vi "UTIL_Add array to queue v1_0_0.vi"(6 "Queue elements":string[](array[string]), 7 "Flush (f)":bool, 8 "error in (no error)":errorcluster, 9 "Queue position":enum16{"top", "bottom"}(ring)=enum."bottom", 11 "Queue in":refnum<queue>) -> (0 "error out":errorcluster, 3 "Queue out":refnum<queue>)   [LabVIEW 2015]
doc: "UTIL_Add array to queue v1_0_0.vi\n\nIf flush queue first boolean is true it revoves any existing queue elements from the queue array. If false, Items already existing on the queue array will remain.\n\nAny items that exist in the Queue elements control are then added to either the top or bottom of the array depending on the Queue position control\n\nCreated 2006 by\nJim Tersigni\nNational Analytics\n970-397-0764"
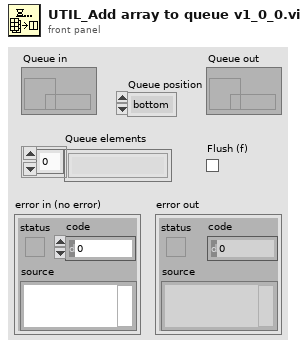
[diagram p1: front panel]
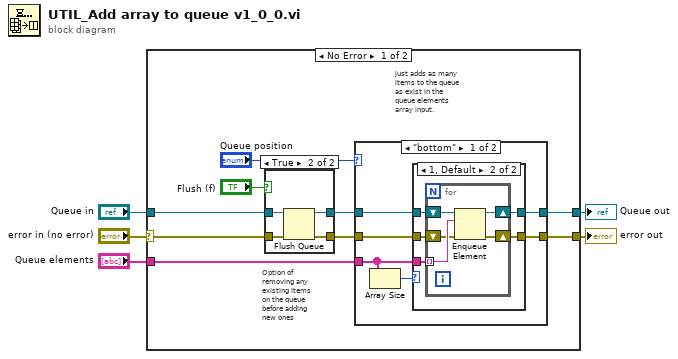
[diagram p0: block diagram]
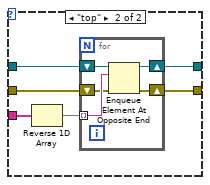
[diagram p4: hidden frame]
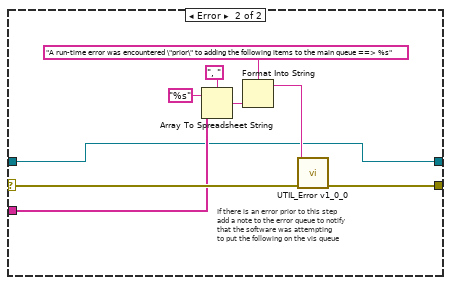
[diagram p5: hidden frame]
diagram:
  n1 = case shown="No Error" "error in (no error)" {
    selector: "error in (no error)" -> [w8 w58]
    tunnel: "Queue in" -> [w14 w51]
    tunnel: [w13 w57] -> w4
    tunnel: "Queue elements" -> [w7 w53]
    tunnel: [w6 w51] -> w1
    frame No Error {
      # "just adds as many\nitems to the queue\nas exist in the\nqueue elements\narray input."
      # "Option of \nremoving any\nexisting items\non the queue\nbefore adding \nnew ones"
      n2 = case shown="True" "Flush (f)" {
        tunnel: w8 -> [w15 w20]
        tunnel: [w15 w19] -> w10
        tunnel: [w16 w18] -> w9
        tunnel: w14 -> [w16 w17]
        frame False {
        }
        frame True {
          n3 = Flush Queue(queue=w17, error in (no error)=w20) -> (queue out=w18:refnum<queue>, error out=w19:errorcluster)  [unwired: 1 out]
        }
      }
      n4 = case shown="\"bottom\"" "Queue position" {
        tunnel: w9 -> [w26 w44]
        tunnel: [w25 w43] -> w6
        tunnel: [w24 w42] -> w13
        tunnel: w10 -> [w23 w41]
        tunnel: w7 -> [w22 w40]
        frame "bottom" {
          n5 = Array Size(array=w22) -> (size(s)=w21:i32)
          n6 = case shown="1, Default" w21 {
            tunnel: w26 -> [w28 w33]
            tunnel: [w28 w32] -> w25
            tunnel: [w27 w31] -> w24
            tunnel: w23 -> [w27 w30]
            tunnel: w22 -> [_ w29]
            frame 0 {
              # "If no items are\nin the control\nthen pass prior\nreference through"
            }
            frame 1, Default {
              n7 = for {
                tunnel: w29 -> [w38] mode=indexing
                shift-right: [w37] -> w32
                shift-left: w33 -> [w36]
                shift-right: [w35] -> w31
                shift-left: w30 -> [w34]
                n8 = Enqueue Element(queue=w36, element=w38, error in (no error)=w34) -> (queue out=w37:refnum<queue>, error out=w35:errorcluster)  [unwired: 2 out]
              }
            }
          }
        }
        frame "top" {
          n9 = Reverse 1D Array(array=w40) -> (reversed array=w39:string[])
          n10 = for {
            tunnel: w39 -> [w49] mode=indexing
            shift-right: [w48] -> w43
            shift-left: w44 -> [w47]
            shift-right: [w46] -> w42
            shift-left: w41 -> [w45]
            n11 = Enqueue Element At Opposite End(queue=w47, element=w49, error in (no error)=w45) -> (queue out=w48:refnum<queue>, error out=w46:errorcluster)  [unwired: 2 out]
          }
        }
      }
    }
    frame Error {
      # "If there is an error prior to this step\nadd a note to the error queue to notify\nthat the software was attempting\nto put the following on the vis queue"
      n12 = Array To Spreadsheet String(delimiter (Tab)=", ", array=w53, 3:"%s" ("format string")) -> (spreadsheet string=w55:string)
      n13 = Format Into String(format string="A run-time error was encountered \"prior\" to adding the following items to the main queue ==> %s", w55) -> (resulting string=w52:string)  [unwired: 2 in, 1 out]
      n14 = call "UTIL_Error v1_0_0.vi"("error in (no error)"=w58, "State"=w52) -> ("error out"=w57:errorcluster)  [unwired: 1 in, 8 out]
    }
  }
  "error out" <- w4
  "Queue out" <- w1
